vi "Fetch Waveform.vi"   [LabVIEW 2012, in "NH Research Regenerative Test Series.lvlib"]
doc: "Return a waveform containing the instantaneous input voltage or current for the specified phase.\n\nWaveforms are captured with every initiated measurement based on the Set Aperture Length.vi and Set Number of Samples.vi commands. A measurement must be initiated first using a Read command or calling Initiate Measurement.vi."
uses:
  <instrlib>/NH Research Regenerative Test Series/NH Research Regenerative Test Series.lvlib
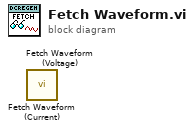
[diagram p0: block diagram]
diagram:
  n1 = call <instrlib>:"Fetch Waveform (Current).vi"() -> ()  [unwired: 13 in, 3 out]
  n2 = call <instrlib>:"Fetch Waveform (Voltage).vi"() -> ()  [unwired: 13 in, 3 out]
